vi "FormatController.vi"() -> ()   [LabVIEW 2014]
panel:
  out "Driver controller 2":T1
  in  "stop":bool
  out "Driver controller":T1
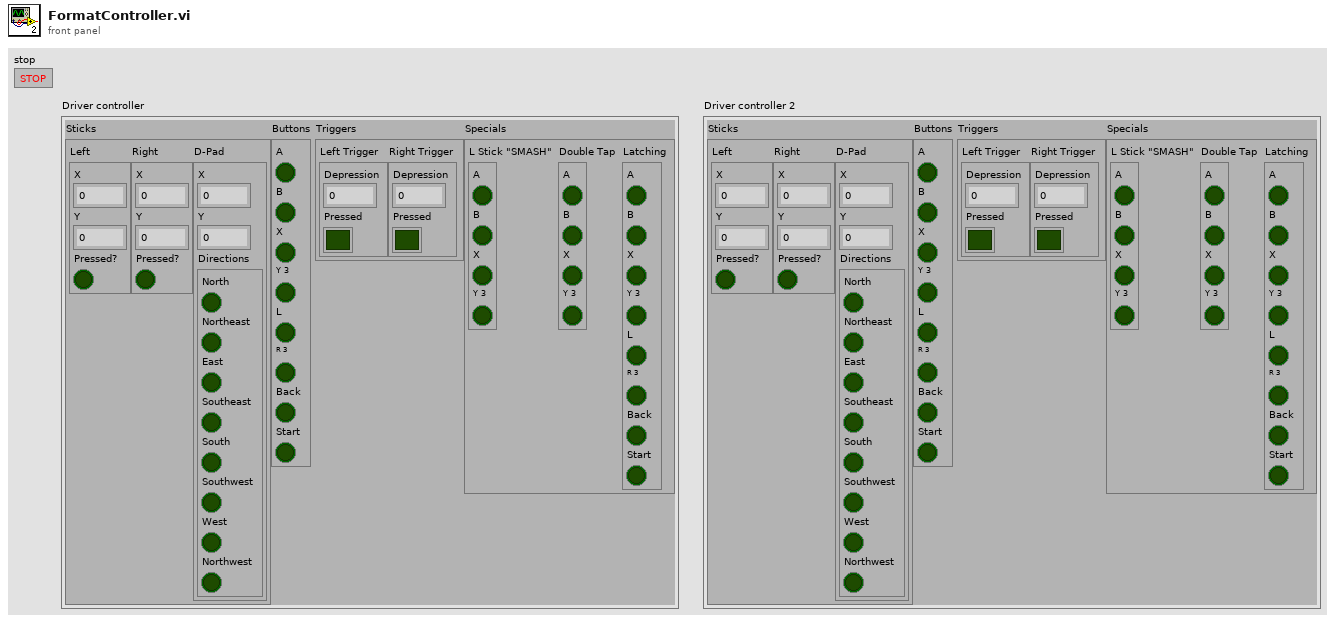
[diagram p1: front panel]
types:
  T1 = cluster{"Sticks":cluster{"Left":cluster{"X":dbl, "Y":dbl, "Pressed?":bool}, "Right":cluster{"X":dbl, "Y":dbl, "Pressed?":bool}, "D-Pad":cluster{"X":dbl, "Y":dbl, "Directions":cluster{"North":bool, "Northeast":bool, "East":bool, "Southeast":bool, "South":bool, "Southwest":bool, "West":bool, "Northwest":bool}}}, "Buttons":cluster{"A":bool, "B":bool, "X":bool, "Y 3":bool, "L":bool, "R 3":bool, "Back":bool, "Start":bool}, "Triggers":cluster{"Left Trigger":cluster{"Depression":dbl, "Pressed":bool}, "Right Trigger":cluster{"Depression":dbl, "Pressed":bool}}, "Specials":cluster{"L Stick \"SMASH\"":cluster{"A":bool, "B":bool, "X":bool, "Y 3":bool}, "Double Tap":cluster{"A":bool, "B":bool, "X":bool, "Y 3":bool}, "Latching":cluster{"A":bool, "B":bool, "X":bool, "Y 3":bool, "L":bool, "R 3":bool, "Back":bool, "Start":bool}}}
  T2 = cluster{"Sticks":cluster{"Left":cluster{"X":dbl, "Y":dbl, "Pressed?":bool}, "Right":cluster{"X":dbl, "Y":dbl, "Pressed?":bool}, "D-Pad":cluster{"X":dbl, "Y":dbl, "Directions":cluster{"North":bool, "Northeast":bool, "East":bool, "Southeast":bool, "South":bool, "Southwest":bool, "West":bool, "Northwest":bool}}}, "Buttons":cluster{"A":bool, "B":bool, "X":bool, "Y 3":bool, "L":bool, "R 3":bool, "Back":bool, "Start":bool}, "Triggers":cluster{"Left Trigger":cluster{"Depression":dbl, "Pressed":bool}, "Right Trigger":cluster{"Depression":dbl, "Pressed":bool}}, "Specials":cluster{"A \"SMASH\"":cluster{"Up":bool, "Down":bool, "Left":bool, "Right 3":bool}, "Double Tap":cluster{"A":bool, "B":bool, "X":bool, "Y 3":bool}, "Latching":cluster{"A":bool, "B":bool, "X":bool, "Y 3":bool, "L":bool, "R 3":bool, "Back":bool, "Start":bool}}}
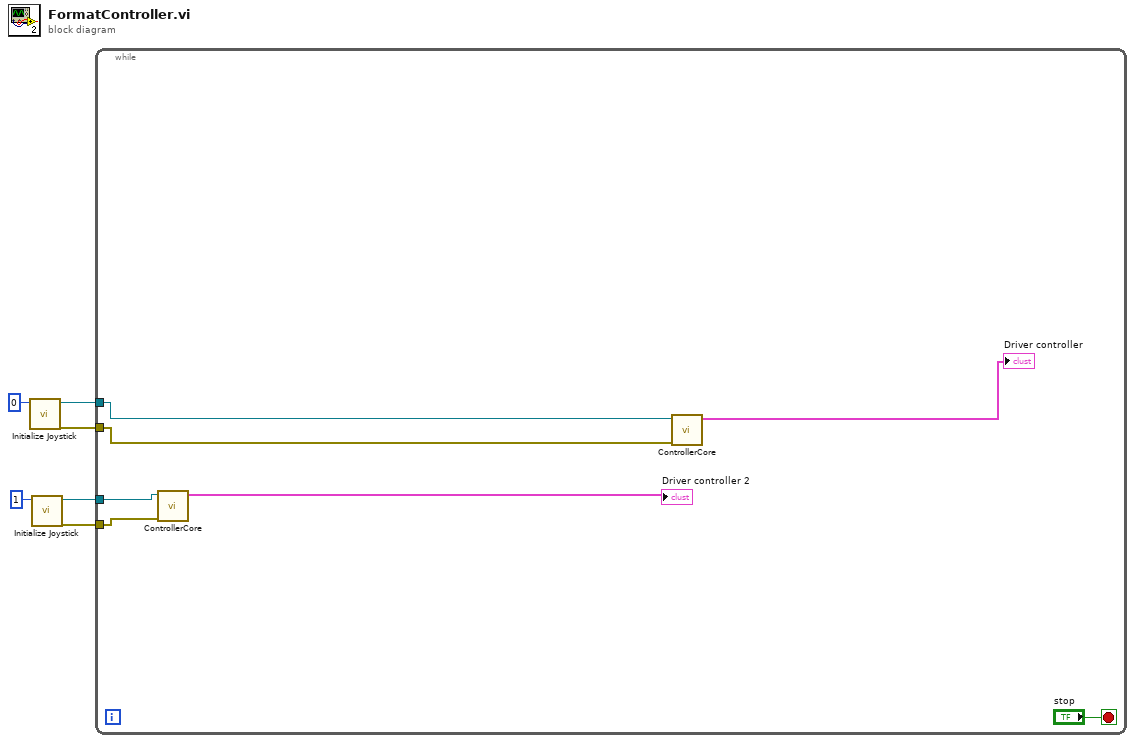
[diagram p0: block diagram]
diagram:
  n1 = call <vilib>:"Initialize Joystick.vi"("device index"=0) -> ("error out"=w5:errorcluster, "device ID"=w6:refnum<k1>)  [unwired: 9 in]
  n2 = call <vilib>:"Initialize Joystick.vi"("device index"=1) -> ("error out"=w2:errorcluster, "device ID"=w1:refnum<k1>)  [unwired: 9 in]
  n3 = while {
    tunnel: w6 -> [w12]
    tunnel: w5 -> [w11]
    tunnel: w1 -> [w9]
    tunnel: w2 -> [w8]
    stop <- "stop" stop-if-true
    n4 = call "ControllerCore.vi"("error in (no error)"=w8, "Refnum in"=w9) -> ("Driver controller"=→"Driver controller 2":T2)  [unwired: 9 in]
    n5 = call "ControllerCore.vi"("error in (no error)"=w11, "Refnum in"=w12) -> ("Driver controller"=→"Driver controller":T2)  [unwired: 9 in]
  }
